vi "cam coerce.vi"(1 "x":dbl) -> (0 "coerced(x)":dbl)   [LabVIEW 2012]
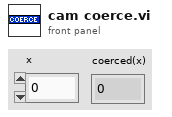
[diagram p1: front panel]
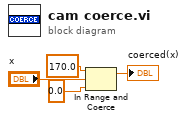
[diagram p0: block diagram]
diagram:
  n1 = In Range and Coerce(upper limit=170.0, x="x", lower limit=0.0) -> (coerced(x)=→"coerced(x)":dbl)  [unwired: 1 out]
